vi "Get Invoke Node Reference.vi"(8 "error in (no error)":errorcluster) -> (0 "error out":errorcluster, 3 "Invoke Refnum":refnum<vi>)   [LabVIEW 2023]
doc: "<b> </b> <b> </b>\n© 2017 Q Software Innovations, LLC\nwritten by Quentin \"Q\" Alldredge\nproduced in LabVIEW 2015\n\nsupport@qsoftwareinnovations.com\nwww.qsoftwareinnovations.com\n\nAll rights reserved.\n\nRedistribution and use in source and binary forms, with or without modification, are permitted provided that the following conditions are met:\n\n * Redistributions of source code must retain the above copyright notice, this list of conditions and the following disclaimer.\n * Redistributions in binary form must reproduce the above copyright notice, this list of conditions and the following disclaimer in the documentation and/or other materials provided with the distribution.\n * Neither the name of Q Software Innovations, LLC. nor the names of its contributors may be used to endorse or promote products derived from this software without specific prior written permission.\n\nTHIS SOFTWARE IS PROVIDED BY THE COPYRIGHT HOLDERS AND CONTRIBUTORS \"AS IS\" AND ANY EXPRESS OR IMPLIED WARRANTIES, INCLUDING, BUT NOT LIMITED TO, THE IMPLIED WARRANTIES OF MERCHANTABILITY AND FITNESS FOR A PARTICULAR PURPOSE ARE DISCLAIMED. IN NO EVENT SHALL THE COPYRIGHT OWNER OR CONTRIBUTORS BE LIABLE FOR ANY DIRECT, INDIRECT, INCIDENTAL, SPECIAL, EXEMPLARY, OR CONSEQUENTIAL DAMAGES (INCLUDING, BUT NOT LIMITED TO, PROCUREMENT OF SUBSTITUTE GOODS OR SERVICES; LOSS OF USE, DATA, OR PROFITS; OR BUSINESS INTERRUPTION) HOWEVER CAUSED AND ON ANY THEORY OF LIABILITY, WHETHER IN CONTRACT, STRICT LIABILITY, OR TORT (INCLUDING NEGLIGENCE OR OTHERWISE) ARISING IN ANY WAY OUT OF THE USE OF THIS SOFTWARE, EVEN IF ADVISED OF THE POSSIBILITY OF SUCH DAMAGE."
uses:
  <vilib>/Utility/traverseref.llb/VI Scripting - Traverse.lvlib
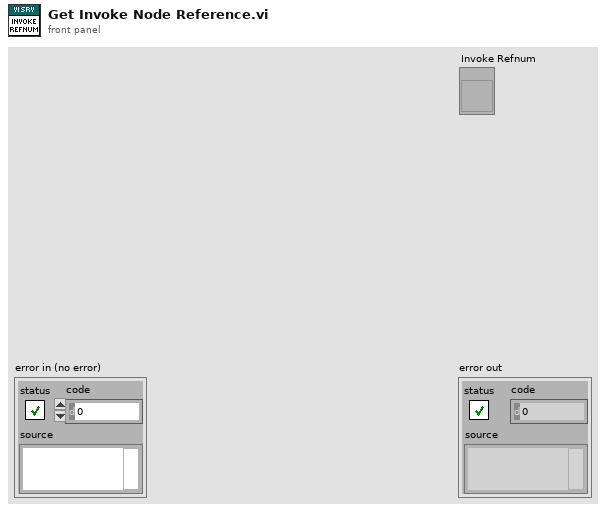
[diagram p1: front panel]
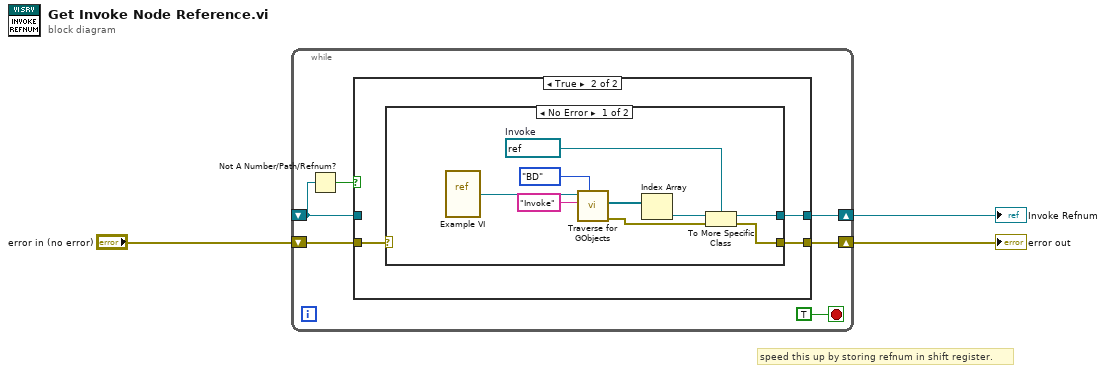
[diagram p0: block diagram]
diagram:
  # "speed this up by storing refnum in shift register."
  n1 = while {
    shift-right: [w8] -> w2
    shift-left: "error in (no error)" -> [w9]
    shift-right: [w7] -> w1
    shift-left: _ -> [w5]
    stop <- TRUE stop-if-true
    n2 = Not A Number/Path/Refnum?(number/path/refnum=w5) -> (NaN/Path/Refnum?=w6:bool)
    n3 = case shown="True" w6 {
      tunnel: w9 -> [w10 w14]
      tunnel: [w10 w13] -> w8
      tunnel: [w11 w12] -> w7
      tunnel: w5 -> [w11 _]
      frame False {
      }
      frame True {
        n4 = case shown="No Error" w14 {
          selector: w14 -> [_ w24]
          tunnel: [w17 w24] -> w13
          tunnel: [w15 _] -> w12
          frame No Error {
            w18 = refnum<vi> refnum  # Invoke
            n5 = vi-ref "Example VI.vi"() -> (w23:refnum<vi>)
            n6 = call <vilib>:"Traverse for GObjects.vi"("Traverse Target"=enum16{"FP", "BD", "Other"}."BD", "Class Name"="Invoke", "VI Refnum"=w23) -> ("error out"=w19:errorcluster, "References"=w21:refnum<vi>[])  [unwired: 5 in, 2 out]
            n7 = Index Array(array=w21) -> (element=w20:refnum<vi>)  [unwired: 1 in]
            n8 = To More Specific Class(target class=w18, reference=w20, error in=w19) -> (specific class reference=w15:refnum<vi>, error out=w17:errorcluster)
          }
          frame Error {
          }
        }
      }
    }
  }
  "error out" <- w2
  "Invoke Refnum" <- w1
